vi "fgv_ctr-ref_gmap.vi"(7 "cmd":T2, 11 "ref in":T1) -> (3 "ref out":T1)   [LabVIEW 2019]
uses:
  Ctrl/cmd_common.ctl
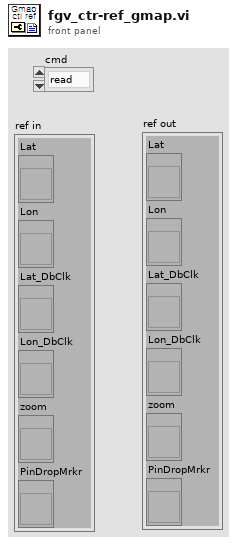
[diagram p1: front panel]
types:
  T1 = cluster{"Lat":refnum<vi>, "Lon":refnum<vi>, "Lat_DbClk":refnum<vi>, "Lon_DbClk":refnum<vi>, "zoom":refnum<vi>, "PinDropMrkr":refnum<vi>}
  T2 = typedef "cmd_common.ctl" = enum16{"read", "write"}
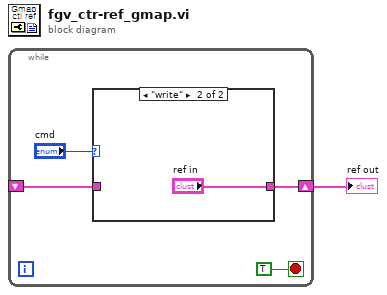
[diagram p0: block diagram]
diagram:
  n1 = while {
    shift-right: [w3] -> w1
    shift-left: _ -> [w2]
    stop <- TRUE stop-if-true
    n2 = case shown="\"write\"" "cmd" {
      tunnel: [w6 "ref in"] -> w3
      tunnel: w2 -> [w6 _]
      frame "read", Default {
      }
      frame "write" {
      }
    }
  }
  "ref out" <- w1
